vi "DataArray_Reformatter.vi"(0 "Data Array":string[][](array[string])) -> (1 "Temps":dbl[][](graph), 2 "FreezeTemps":dbl[](array[numeric]), 3 "Offsets":dbl[](array[numeric]), 4 "Offset Applied":bool)   [LabVIEW 2020]
panel:
  out "Array":dbl[][](array[numeric])
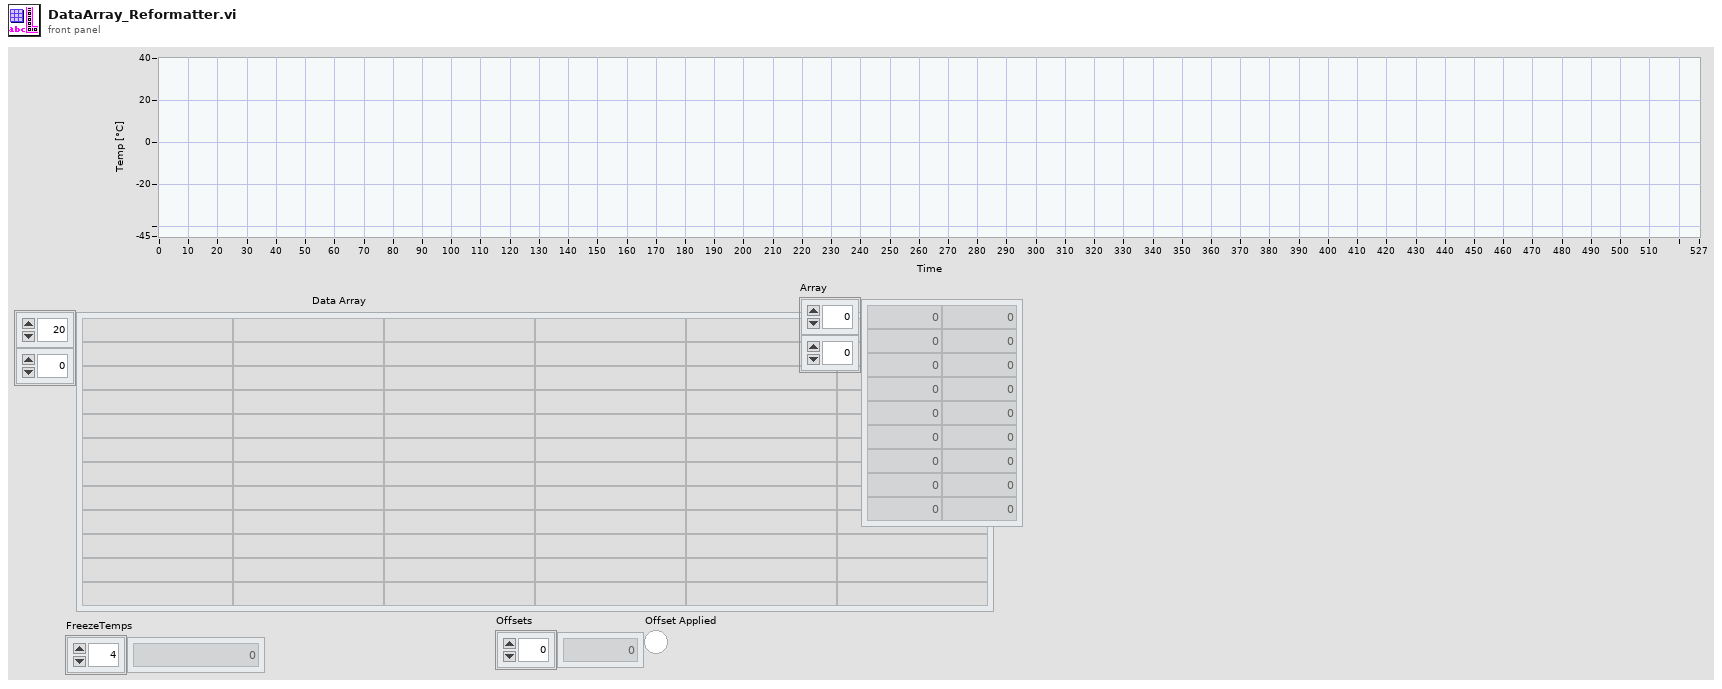
[diagram p1: front panel]
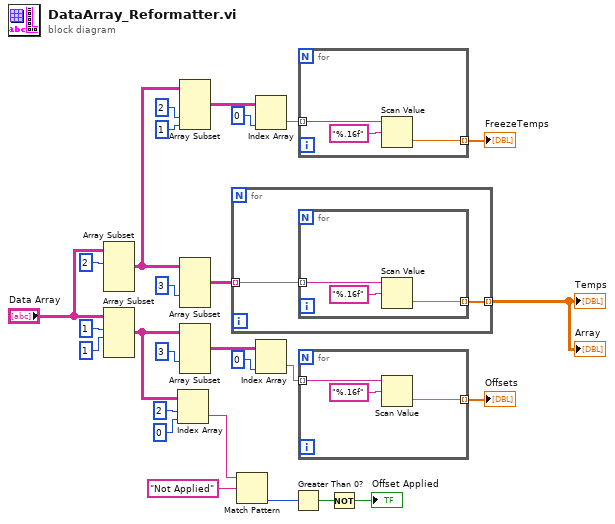
[diagram p0: block diagram]
diagram:
  n1 = Array Subset(array="Data Array", index (row)=2 ("index")) -> (w24:string[][])  [unwired: 3 in]
  n2 = Array Subset(array="Data Array", index (row)=1 ("index"), length (row)=1 ("length")) -> (w13:string[][])  [unwired: 2 in]
  n3 = Index Array(array=w13, index (row)=2, index (col)=0 ("disabled index (col)")) -> (element=w5:string)
  n4 = Array Subset(array=w24, index (col)=2 ("index"), length (col)=1 ("length")) -> (w25:string[][])  [unwired: 2 in]
  n5 = Array Subset(array=w24, index (col)=3 ("index")) -> (w20:string[][])  [unwired: 3 in]
  n6 = Array Subset(array=w13, index (col)=3 ("index")) -> (w11:string[][])  [unwired: 3 in]
  n7 = for {
    tunnel: w20 -> [w29] mode=indexing
    tunnel: [w28] -> w19 mode=indexing
    n8 = for {
      tunnel: w29 -> [w31] mode=indexing
      tunnel: [w30] -> w28 mode=indexing
      n9 = Scan Value(string=w31, format string="%.16f") -> (value=w30:dbl)  [unwired: 1 in, 1 out]
    }
  }
  "Temps" <- w19
  "Array" <- w19
  n10 = Match Pattern(string=w5, regular expression="Not Applied") -> (offset past match=w3:i32)  [unwired: 1 in, 3 out]
  n11 = Index Array(array=w25, index (col)=0 ("disabled index (col)")) -> (element=w18:string[])  [unwired: 1 in]
  n12 = Index Array(array=w11, index (col)=0 ("disabled index (col)")) -> (element=w9:string[])  [unwired: 1 in]
  n13 = Greater Than 0?(x=w3) -> (x > 0?=w2:bool)
  n14 = for {
    tunnel: w18 -> [w34] mode=indexing
    tunnel: [w33] -> w17 mode=indexing
    n15 = Scan Value(string=w34, format string="%.16f") -> (value=w33:dbl)  [unwired: 1 in, 1 out]
  }
  "FreezeTemps" <- w17
  n16 = for {
    tunnel: w9 -> [w37] mode=indexing
    tunnel: [w36] -> w8 mode=indexing
    n17 = Scan Value(string=w37, format string="%.16f") -> (value=w36:dbl)  [unwired: 1 in, 1 out]
  }
  "Offsets" <- w8
  n18 = Not(x=w2) -> (.not. x?=→"Offset Applied":bool)
